vi "AnalogDemultiplex_AND_drop_first_two_samples.vi"(0 "Analog data cluster":T1, 5 "Over? Array":bool[](array[boolean])=[FALSE, FALSE, FALSE, FALSE, FALSE, FALSE, FALSE, FALSE], 7 "Last Sample A1":u8, 9 "Last Sample A2":u8, 11 "Last? Input":bool) -> (4 "Data A1 out":u64, 6 "Data A2 out":u64, 15 "Last? Output":bool)   [LabVIEW 2012]
panel:
  out "Wrap Output":bool
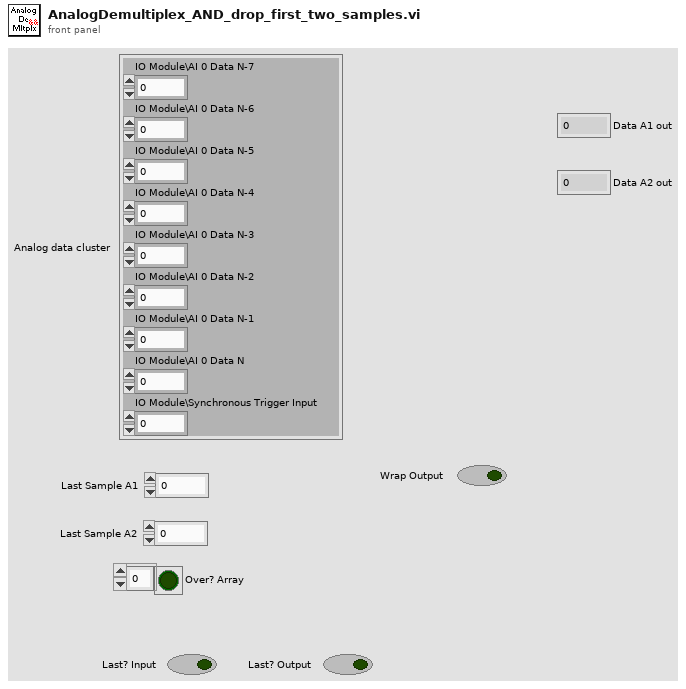
[diagram p1: front panel]
types:
  T1 = cluster{"IO Module\\AI 0 Data N-7":u8, "IO Module\\AI 0 Data N-6":u8, "IO Module\\AI 0 Data N-5":u8, "IO Module\\AI 0 Data N-4":u8, "IO Module\\AI 0 Data N-3":u8, "IO Module\\AI 0 Data N-2":u8, "IO Module\\AI 0 Data N-1":u8, "IO Module\\AI 0 Data N":u8, "IO Module\\Synchronous Trigger Input":u8}
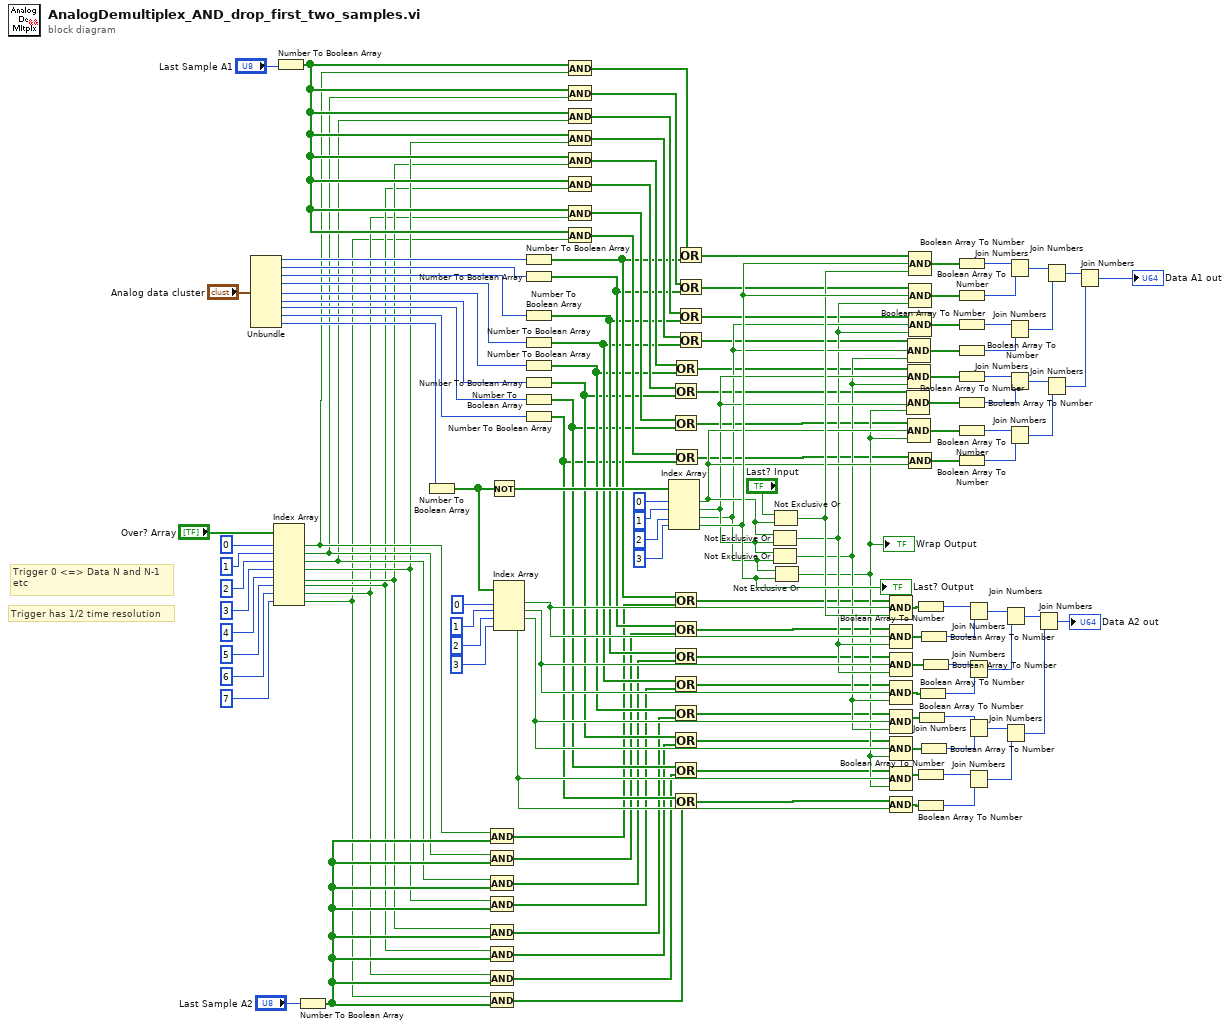
[diagram p0: block diagram]
diagram:
  # "Trigger 0 <=> Data N and N-1\netc"
  # "Trigger has 1/2 time resolution"
  n1 = Unbundle("Analog data cluster") -> ("IO Module\\AI 0 Data N-7"=w102:u8, "IO Module\\AI 0 Data N-6"=w101:u8, "IO Module\\AI 0 Data N-5"=w100:u8, "IO Module\\AI 0 Data N-4"=w99:u8, "IO Module\\AI 0 Data N-3"=w98:u8, "IO Module\\AI 0 Data N-2"=w97:u8, "IO Module\\AI 0 Data N-1"=w96:u8, "IO Module\\AI 0 Data N"=w95:u8, "IO Module\\Synchronous Trigger Input"=w94:u8)
  n2 = Index Array(array="Over? Array", index #1=0 ("index"), index #2=1 ("index"), index #3=2 ("index"), index #4=3 ("index"), index #5=4 ("index"), index #6=5 ("index"), index #7=6 ("index"), index #8=7 ("index")) -> (element #1=w48:bool, element #2=w47:bool, element #3=w46:bool, element #4=w45:bool, element #5=w44:bool, element #6=w43:bool, element #7=w42:bool, element #8=w41:bool)
  n3 = Number To Boolean Array(number="Last Sample A1") -> (Boolean array=w50:bool[])
  n4 = Number To Boolean Array(number="Last Sample A2") -> (Boolean array=w49:bool[])
  n5 = Number To Boolean Array(number=w94) -> (Boolean array=w66:bool[])
  n6 = And(x=w48, y=w49) -> (x .and. y?=w8:bool[])
  n7 = And(x=w47, y=w49) -> (x .and. y?=w7:bool[])
  n8 = And(x=w46, y=w49) -> (x .and. y?=w6:bool[])
  n9 = And(x=w45, y=w49) -> (x .and. y?=w5:bool[])
  n10 = And(x=w44, y=w49) -> (x .and. y?=w1:bool[])
  n11 = And(x=w43, y=w49) -> (x .and. y?=w2:bool[])
  n12 = And(x=w42, y=w49) -> (x .and. y?=w3:bool[])
  n13 = And(x=w41, y=w49) -> (x .and. y?=w4:bool[])
  n14 = Not(x=w66) -> (.not. x?=w65:bool[])
  n15 = Index Array(array=w66, index #1=0 ("index"), index #2=1 ("index"), index #3=2 ("index"), index #4=3 ("index")) -> (element #1=w74:bool, element #2=w77:bool, element #3=w79:bool, element #4=w81:bool)
  n16 = Number To Boolean Array(number=w102) -> (Boolean array=w24:bool[])
  n17 = Number To Boolean Array(number=w101) -> (Boolean array=w23:bool[])
  n18 = Number To Boolean Array(number=w100) -> (Boolean array=w22:bool[])
  n19 = Number To Boolean Array(number=w99) -> (Boolean array=w21:bool[])
  n20 = Number To Boolean Array(number=w98) -> (Boolean array=w20:bool[])
  n21 = Number To Boolean Array(number=w97) -> (Boolean array=w19:bool[])
  n22 = Number To Boolean Array(number=w96) -> (Boolean array=w18:bool[])
  n23 = Number To Boolean Array(number=w95) -> (Boolean array=w17:bool[])
  n24 = And(x=w50, y=w48) -> (x .and. y?=w25:bool[])
  n25 = And(x=w50, y=w47) -> (x .and. y?=w26:bool[])
  n26 = And(x=w50, y=w46) -> (x .and. y?=w27:bool[])
  n27 = And(x=w50, y=w45) -> (x .and. y?=w28:bool[])
  n28 = And(x=w50, y=w44) -> (x .and. y?=w29:bool[])
  n29 = And(x=w50, y=w43) -> (x .and. y?=w30:bool[])
  n30 = And(x=w50, y=w42) -> (x .and. y?=w31:bool[])
  n31 = And(x=w50, y=w41) -> (x .and. y?=w32:bool[])
  n32 = Index Array(array=w65, index #1=0 ("index"), index #2=1 ("index"), index #3=2 ("index"), index #4=3 ("index")) -> (element #1=w72:bool, element #2=w70:bool, element #3=w68:bool, element #4=w83:bool)
  "Last? Output" <- w83
  n33 = Or(x=w30, y=w19) -> (x .or. y?=w38:bool[])
  n34 = Or(x=w31, y=w18) -> (x .or. y?=w39:bool[])
  n35 = Or(x=w24, y=w8) -> (x .or. y?=w16:bool[])
  n36 = Or(x=w23, y=w7) -> (x .or. y?=w15:bool[])
  n37 = Or(x=w22, y=w6) -> (x .or. y?=w14:bool[])
  n38 = Or(x=w21, y=w5) -> (x .or. y?=w13:bool[])
  n39 = Or(x=w20, y=w1) -> (x .or. y?=w12:bool[])
  n40 = Or(x=w19, y=w2) -> (x .or. y?=w11:bool[])
  n41 = Or(x=w18, y=w3) -> (x .or. y?=w10:bool[])
  n42 = Or(x=w17, y=w4) -> (x .or. y?=w9:bool[])
  n43 = Or(x=w29, y=w20) -> (x .or. y?=w37:bool[])
  n44 = Or(x=w32, y=w17) -> (x .or. y?=w40:bool[])
  n45 = Or(x=w25, y=w24) -> (x .or. y?=w33:bool[])
  n46 = Or(x=w26, y=w23) -> (x .or. y?=w34:bool[])
  n47 = Or(x=w27, y=w22) -> (x .or. y?=w35:bool[])
  n48 = Or(x=w28, y=w21) -> (x .or. y?=w36:bool[])
  n49 = Not Exclusive Or(1:w70, 2:w72) -> (0:w64:bool)
  n50 = Not Exclusive Or(1:w68, 2:w70) -> (0:w63:bool)
  n51 = Not Exclusive Or(1:w72, 2:"Last? Input") -> (0:w75:bool)
  n52 = Not Exclusive Or(1:w83, 2:w68) -> (0:w62:bool)
  "Wrap Output" <- w62
  n53 = Compound Arithmetic op=AND(w16, w74, w75) -> (w135:bool[])
  n54 = Compound Arithmetic op=AND(w15, w74, w64) -> (w73:bool[])
  n55 = Compound Arithmetic op=AND(w14, w77, w64) -> (w136:bool[])
  n56 = Compound Arithmetic op=AND(w13, w77, w63) -> (w76:bool[])
  n57 = Compound Arithmetic op=AND(w12, w79, w63) -> (w137:bool[])
  n58 = Compound Arithmetic op=AND(w11, w79, w62) -> (w78:bool[])
  n59 = Compound Arithmetic op=AND(w10, w81, w62) -> (w138:bool[])
  n60 = Compound Arithmetic op=AND(w9, w81) -> (w80:bool[])
  n61 = Compound Arithmetic op=AND(w38, w70, w62) -> (w69:bool[])
  n62 = Compound Arithmetic op=AND(w36, w68, w63) -> (w67:bool[])
  n63 = Compound Arithmetic op=AND(w37, w70, w63) -> (w112:bool[])
  n64 = Compound Arithmetic op=AND(w39, w72, w62) -> (w113:bool[])
  n65 = Compound Arithmetic op=AND(w33, w83, w75) -> (w109:bool[])
  n66 = Compound Arithmetic op=AND(w34, w83, w64) -> (w82:bool[])
  n67 = Compound Arithmetic op=AND(w35, w68, w64) -> (w111:bool[])
  n68 = Compound Arithmetic op=AND(w40, w72) -> (w71:bool[])
  n69 = Boolean Array To Number(Boolean array=w135) -> (number=w127:u8)
  n70 = Boolean Array To Number(Boolean array=w138) -> (number=w133:u8)
  n71 = Boolean Array To Number(Boolean array=w80) -> (number=w134:u8)
  n72 = Boolean Array To Number(Boolean array=w137) -> (number=w131:u8)
  n73 = Boolean Array To Number(Boolean array=w76) -> (number=w130:u8)
  n74 = Boolean Array To Number(Boolean array=w73) -> (number=w128:u8)
  n75 = Boolean Array To Number(Boolean array=w78) -> (number=w132:u8)
  n76 = Boolean Array To Number(Boolean array=w136) -> (number=w129:u8)
  n77 = Boolean Array To Number(Boolean array=w109) -> (number=w110:u8)
  n78 = Boolean Array To Number(Boolean array=w82) -> (number=w114:u8)
  n79 = Boolean Array To Number(Boolean array=w111) -> (number=w115:u8)
  n80 = Boolean Array To Number(Boolean array=w67) -> (number=w116:u8)
  n81 = Boolean Array To Number(Boolean array=w112) -> (number=w117:u8)
  n82 = Boolean Array To Number(Boolean array=w69) -> (number=w118:u8)
  n83 = Boolean Array To Number(Boolean array=w113) -> (number=w119:u8)
  n84 = Boolean Array To Number(Boolean array=w71) -> (number=w120:u8)
  n85 = Join Numbers(hi=w127, lo=w128) -> ((hi.lo)=w121:u16)
  n86 = Join Numbers(hi=w129, lo=w130) -> ((hi.lo)=w122:u16)
  n87 = Join Numbers(hi=w131, lo=w132) -> ((hi.lo)=w123:u16)
  n88 = Join Numbers(hi=w133, lo=w134) -> ((hi.lo)=w124:u16)
  n89 = Join Numbers(hi=w121, lo=w122) -> ((hi.lo)=w126:u32)
  n90 = Join Numbers(hi=w123, lo=w124) -> ((hi.lo)=w125:u32)
  n91 = Join Numbers(hi=w110, lo=w114) -> ((hi.lo)=w103:u16)
  n92 = Join Numbers(hi=w115, lo=w116) -> ((hi.lo)=w104:u16)
  n93 = Join Numbers(hi=w117, lo=w118) -> ((hi.lo)=w105:u16)
  n94 = Join Numbers(hi=w119, lo=w120) -> ((hi.lo)=w106:u16)
  n95 = Join Numbers(hi=w126, lo=w125) -> ((hi.lo)=→"Data A2 out":u64)
  n96 = Join Numbers(hi=w103, lo=w104) -> ((hi.lo)=w108:u32)
  n97 = Join Numbers(hi=w105, lo=w106) -> ((hi.lo)=w107:u32)
  n98 = Join Numbers(hi=w108, lo=w107) -> ((hi.lo)=→"Data A1 out":u64)
